vi "Synth Enter Zeros.vi"(8 "Error In":errorcluster, 11 "DAQmx Device Name":tag) -> (0 "Error Out":errorcluster, 3 "DAQmx Device Name out":tag)   [LabVIEW 2016]
uses:
  <vilib>/DAQmx/write.llb/DAQmx Write (Digital U8 1Chan 1Samp).vi
  <vilib>/DAQmx/create/channels.llb/DAQmx Create Channel (DO-Digital Output).vi
  <vilib>/DAQmx/miscellaneous.llb/DAQmx Fill In Error Info.vi
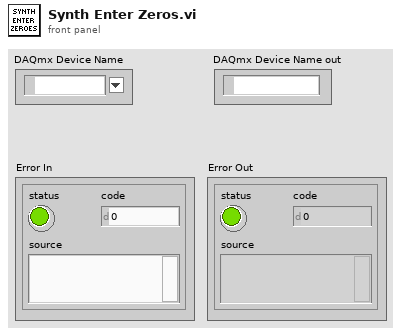
[diagram p1: front panel]
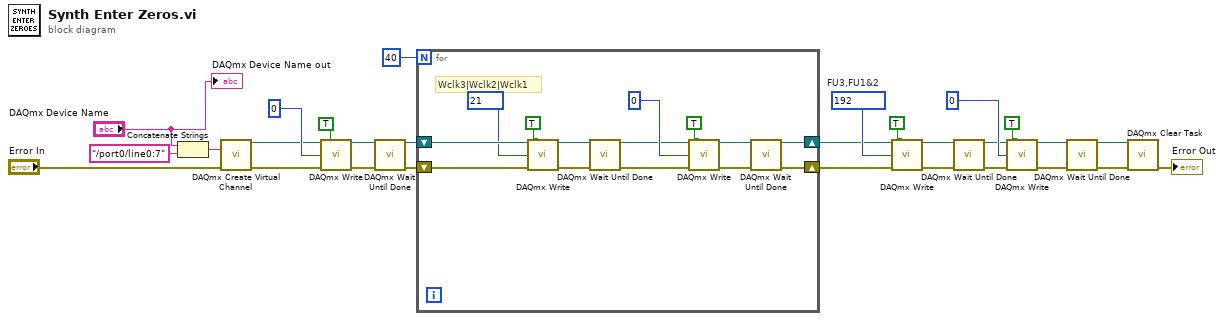
[diagram p0: block diagram]
diagram:
  w16 = u8 192  # FU3,FU1&2
  n1 = Concatenate Strings("DAQmx Device Name", "/port0/line0:7") -> (w5:string)
  n2 = call-poly <vilib>:"DAQmx Create Virtual Channel.vi"("lines"=w5, "error in"="Error In") -> ("task out"=w22:refnum<k21>, "error out"=w28:errorcluster)  [unwired: 3 in, 9 out]
  n3 = call-poly <vilib>:"DAQmx Write.vi"("task/channels in"=w22, "auto start"=TRUE, "data"=u8 0, "error in"=w28) -> ("task out"=w21:refnum<k21>, "error out"=w27:errorcluster)  [unwired: 10 out]
  n4 = call <vilib>:"DAQmx Wait Until Done.vi"("task/channels in"=w21, "error in"=w27) -> ("task out"=w20:refnum<k21>, "error out"=w23:errorcluster)  [unwired: 1 in, 11 out]
  n5 = for {
    N: 40 -> [_]
    shift-right: [w29] -> w6
    shift-left: w23 -> [w42]
    shift-right: [w30] -> w7
    shift-left: w20 -> [w41]
    # "Wclk3|Wclk2|Wclk1"
    n6 = call-poly <vilib>:"DAQmx Write.vi"("task/channels in"=w41, "auto start"=TRUE, "data"=21 ("Waveform"), "error in"=w42) -> ("task out"=w38:refnum<k21>, "error out"=w40:errorcluster)  [unwired: 10 out]
    n7 = call <vilib>:"DAQmx Wait Until Done.vi"("task/channels in"=w38, "error in"=w40) -> ("task out"=w32:refnum<k21>, "error out"=w31:errorcluster)  [unwired: 1 in, 11 out]
    n8 = call-poly <vilib>:"DAQmx Write.vi"("task/channels in"=w32, "auto start"=TRUE, "data"=u8 0 ("Waveform"), "error in"=w31) -> ("task out"=w34:refnum<k21>, "error out"=w36:errorcluster)  [unwired: 10 out]
    n9 = call <vilib>:"DAQmx Wait Until Done.vi"("task/channels in"=w34, "error in"=w36) -> ("task out"=w30:refnum<k21>, "error out"=w29:errorcluster)  [unwired: 1 in, 11 out]
  }
  n10 = call-poly <vilib>:"DAQmx Write.vi"("task/channels in"=w7, "auto start"=TRUE, "data"=w16, "error in"=w6) -> ("task out"=w17:refnum<k21>, "error out"=w19:errorcluster)  [unwired: 10 out]
  n11 = call <vilib>:"DAQmx Wait Until Done.vi"("task/channels in"=w17, "error in"=w19) -> ("task out"=w11:refnum<k21>, "error out"=w10:errorcluster)  [unwired: 1 in, 11 out]
  n12 = call-poly <vilib>:"DAQmx Write.vi"("task/channels in"=w11, "auto start"=TRUE, "data"=u8 0 ("Waveform"), "error in"=w10) -> ("task out"=w13:refnum<k21>, "error out"=w15:errorcluster)  [unwired: 10 out]
  n13 = call <vilib>:"DAQmx Wait Until Done.vi"("task/channels in"=w13, "error in"=w15) -> ("task out"=w8:refnum<k21>, "error out"=w9:errorcluster)  [unwired: 1 in, 11 out]
  n14 = call <vilib>:"DAQmx Clear Task.vi"("task in"=w8, "error in"=w9) -> ("error out"=→"Error Out":errorcluster)  [unwired: 13 out]
  "DAQmx Device Name out" <- "DAQmx Device Name"
